vi "SPI Master with debug [Host].vi"() -> ()   [LabVIEW 2019]
uses:
  <vilib>/rvi/interface/RandomDataEmulation/nirviRandomDataOpen.vi
  <vilib>/rvi/interface/common/niFpgaCacheSessionInfoDynamic.vi
  <vilib>/Utility/error.llb/Error Cluster From Error Code.vi
  <vilib>/rvi/errors/niLvFpgaAdjustHostInterfaceError.vi
  <vilib>/Waveform/DWDTOps.llb/DWDT Binary U8 to Digital.vi
  <vilib>/Waveform/DWDTOps.llb/DWDT Binary U32 to Digital.vi
  <vilib>/FPGAPlugInAG/Dynamic/niLvFpga_Close_Dynamic.vi
  <vilib>/rvi/interface/nirviOpenFPGA/nirviOpenFPGA.xnode
  SPI Master with debug [FPGA].vi
  <vilib>/rvi/interface/nirviReadWriteControl/nirviReadWriteControl.xnode
  <vilib>/rvi/interface/nirviMethod/nirviMethod.xnode
  <vilib>/rvi/interface/nirviCloseFPGA/nirviCloseFPGA.xnode
  NiFpgaLv.dll
  <vilib>/rvi/interface/Simulation/niFpgaSimulationCallBeginRW.vi
  <vilib>/FPGAPlugInAG/Dynamic/niLvFpga_ReadFifo_Dynamic.vi
  <vilib>/rvi/errors/niLvFpgaMergeErrorWithErrorCode.vi
panel:
  in  "CPOL":bool
  in  "CPHA":bool
  in  "Data Length":u8=16
  in  "Data In":u32=2779077210 format="%x"
  out "Digital Waveform Graph":digitalwaveform[](graph)=[{"t0"=timestamp(0 s since 1904-01-01), "dt"=1e-08, "Y"={"transitions"=[0, 1, 2, 3, 4, 5, 6, 7, 8, 9, 10, 11, 12, 13, 14, 15, 16, 17, 18, 19, 20, 21, 22, 23, 24, 25, 26, 27, 28, 29, 30, 31, 32, 33, 99], "data"=[[0, 0, 0, 0, 0, 0, 1, 0], [0, 0, 0, 0, 0, 1, 0, 0], [0, 0, 0, 0, 0, 1, 0, 1], [0, 0, 0, 0, 0, 1, 0, 0], [0, 0, 0, 0, 0, 1, 0, 1], [0, 0, 0, 0, 0, 1, 0, 0], [0, 0, 0, 0, 0, 1, 0, 1], [0, 0, 0, 0, 0, 1, 0, 0], [0, 0, 0, 0, 0, 1, 0, 1], [0, 0, 0, 0, 0, 1, 0, 0], [0, 0, 0, 0, 0, 1, 0, 1], [0, 0, 0, 0, 0, 1, 0, 0], [0, 0, 0, 0, 0, 1, 0, 1], [0, 0, 0, 0, 0, 1, 0, 0], [0, 0, 0, 0, 0, 1, 0, 1], [0, 0, 0, 0, 0, 1, 0, 0], [0, 0, 0, 0, 0, 1, 0, 1], [0, 0, 0, 0, 0, 1, 0, 0], [0, 0, 0, 0, 0, 1, 0, 1], [0, 0, 0, 0, 0, 1, 0, 0], [0, 0, 0, 0, 0, 1, 0, 1], [0, 0, 0, 0, 0, 1, 0, 0], [0, 0, 0, 0, 0, 1, 0, 1], [0, 0, 0, 0, 0, 1, 0, 0], [0, 0, 0, 0, 0, 1, 0, 1], [0, 0, 0, 0, 0, 1, 0, 0], [0, 0, 0, 0, 0, 1, 0, 1], [0, 0, 0, 0, 0, 1, 0, 0], [0, 0, 0, 0, 0, 1, 0, 1], [0, 0, 0, 0, 0, 1, 0, 0], [0, 0, 0, 0, 0, 1, 0, 1], [0, 0, 0, 0, 0, 1, 0, 0], [0, 0, 0, 0, 0, 0, 1, 1], [0, 0, 0, 0, 0, 0, 0, 1], [0, 0, 0, 0, 0, 0, 0, 1]]}}, {"t0"=timestamp(0 s since 1904-01-01), "dt"=1e-08, "Y"={"transitions"=[0, 1, 2, 3, 4, 5, 6, 7, 8, 9, 10, 11, 12, 13, 14, 15, 16, 17, 18, 19, 20, 21, 22, 23, 24, 25, 26, 27, 28, 29, 30, 31, 32, 33, 34, 99], "data"=[[0, 0, 0, 0, 1, 0, 0, 0], [0, 0, 1, 0, 0, 0, 0, 0], [0, 0, 1, 1, 0, 0, 0, 0], [0, 0, 0, 0, 0, 0, 0, 0], [0, 0, 0, 1, 0, 0, 0, 0], [0, 0, 1, 0, 0, 0, 0, 0], [0, 0, 1, 1, 0, 0, 0, 0], [0, 0, 0, 0, 0, 0, 0, 0], [0, 0, 0, 1, 0, 0, 0, 0], [0, 0, 0, 0, 0, 0, 0, 0], [0, 0, 0, 1, 0, 0, 0, 0], [0, 0, 1, 0, 0, 0, 0, 0], [0, 0, 1, 1, 0, 0, 0, 0], [0, 0, 0, 0, 0, 0, 0, 0], [0, 0, 0, 1, 0, 0, 0, 0], [0, 0, 1, 0, 0, 0, 0, 0], [0, 0, 1, 1, 0, 0, 0, 0], [0, 0, 1, 0, 0, 0, 0, 0], [0, 0, 1, 1, 0, 0, 0, 0], [0, 0, 0, 0, 0, 0, 0, 0], [0, 0, 0, 1, 0, 0, 0, 0], [0, 0, 1, 0, 0, 0, 0, 0], [0, 0, 1, 1, 0, 0, 0, 0], [0, 0, 0, 0, 0, 0, 0, 0], [0, 0, 0, 1, 0, 0, 0, 0], [0, 0, 0, 0, 0, 0, 0, 0], [0, 0, 0, 1, 0, 0, 0, 0], [0, 0, 1, 0, 0, 0, 0, 0], [0, 0, 1, 1, 0, 0, 0, 0], [0, 0, 0, 0, 0, 0, 0, 0], [0, 0, 0, 1, 0, 0, 0, 0], [0, 0, 1, 0, 0, 0, 0, 0], [0, 0, 1, 1, 0, 0, 0, 0], [0, 0, 1, 0, 0, 0, 0, 0], [0, 0, 1, 0, 1, 0, 0, 0], [0, 0, 1, 0, 1, 0, 0, 0]]}}, {"t0"=timestamp(0 s since 1904-01-01), "dt"=1e-08, "Y"={"transitions"=[0, 1, 3, 5, 7, 9, 11, 13, 15, 17, 19, 21, 23, 25, 27, 29, 31, 99], "data"=[[1, 0, 1, 0, 0, 1, 0, 1, 1, 0, 1, 0, 0, 1, 0, 1, 0, 1, 0, 1, 1, 0, 1, 0, 0, 1, 0, 1, 1, 0, 1, 0], [0, 1, 0, 0, 1, 0, 1, 1, 0, 1, 0, 0, 1, 0, 1, 0, 1, 0, 1, 1, 0, 1, 0, 0, 1, 0, 1, 1, 0, 1, 0, 0], [1, 0, 0, 1, 0, 1, 1, 0, 1, 0, 0, 1, 0, 1, 0, 1, 0, 1, 1, 0, 1, 0, 0, 1, 0, 1, 1, 0, 1, 0, 0, 0], [0, 0, 1, 0, 1, 1, 0, 1, 0, 0, 1, 0, 1, 0, 1, 0, 1, 1, 0, 1, 0, 0, 1, 0, 1, 1, 0, 1, 0, 0, 0, 0], [0, 1, 0, 1, 1, 0, 1, 0, 0, 1, 0, 1, 0, 1, 0, 1, 1, 0, 1, 0, 0, 1, 0, 1, 1, 0, 1, 0, 0, 0, 0, 0], [1, 0, 1, 1, 0, 1, 0, 0, 1, 0, 1, 0, 1, 0, 1, 1, 0, 1, 0, 0, 1, 0, 1, 1, 0, 1, 0, 0, 0, 0, 0, 0], [0, 1, 1, 0, 1, 0, 0, 1, 0, 1, 0, 1, 0, 1, 1, 0, 1, 0, 0, 1, 0, 1, 1, 0, 1, 0, 0, 0, 0, 0, 0, 0], [1, 1, 0, 1, 0, 0, 1, 0, 1, 0, 1, 0, 1, 1, 0, 1, 0, 0, 1, 0, 1, 1, 0, 1, 0, 0, 0, 0, 0, 0, 0, 0], [1, 0, 1, 0, 0, 1, 0, 1, 0, 1, 0, 1, 1, 0, 1, 0, 0, 1, 0, 1, 1, 0, 1, 0, 0, 0, 0, 0, 0, 0, 0, 0], [0, 1, 0, 0, 1, 0, 1, 0, 1, 0, 1, 1, 0, 1, 0, 0, 1, 0, 1, 1, 0, 1, 0, 0, 0, 0, 0, 0, 0, 0, 0, 0], [1, 0, 0, 1, 0, 1, 0, 1, 0, 1, 1, 0, 1, 0, 0, 1, 0, 1, 1, 0, 1, 0, 0, 0, 0, 0, 0, 0, 0, 0, 0, 0], [0, 0, 1, 0, 1, 0, 1, 0, 1, 1, 0, 1, 0, 0, 1, 0, 1, 1, 0, 1, 0, 0, 0, 0, 0, 0, 0, 0, 0, 0, 0, 0], [0, 1, 0, 1, 0, 1, 0, 1, 1, 0, 1, 0, 0, 1, 0, 1, 1, 0, 1, 0, 0, 0, 0, 0, 0, 0, 0, 0, 0, 0, 0, 0], [1, 0, 1, 0, 1, 0, 1, 1, 0, 1, 0, 0, 1, 0, 1, 1, 0, 1, 0, 0, 0, 0, 0, 0, 0, 0, 0, 0, 0, 0, 0, 0], [0, 1, 0, 1, 0, 1, 1, 0, 1, 0, 0, 1, 0, 1, 1, 0, 1, 0, 0, 0, 0, 0, 0, 0, 0, 0, 0, 0, 0, 0, 0, 0], [1, 0, 1, 0, 1, 1, 0, 1, 0, 0, 1, 0, 1, 1, 0, 1, 0, 0, 0, 0, 0, 0, 0, 0, 0, 0, 0, 0, 0, 0, 0, 0], [0, 1, 0, 1, 1, 0, 1, 0, 0, 1, 0, 1, 1, 0, 1, 0, 0, 0, 0, 0, 0, 0, 0, 0, 0, 0, 0, 0, 0, 0, 0, 0], [0, 1, 0, 1, 1, 0, 1, 0, 0, 1, 0, 1, 1, 0, 1, 0, 0, 0, 0, 0, 0, 0, 0, 0, 0, 0, 0, 0, 0, 0, 0, 0]]}}]
  in  "Stop Simulation":bool
  in  "Simulation Steps":u32=100
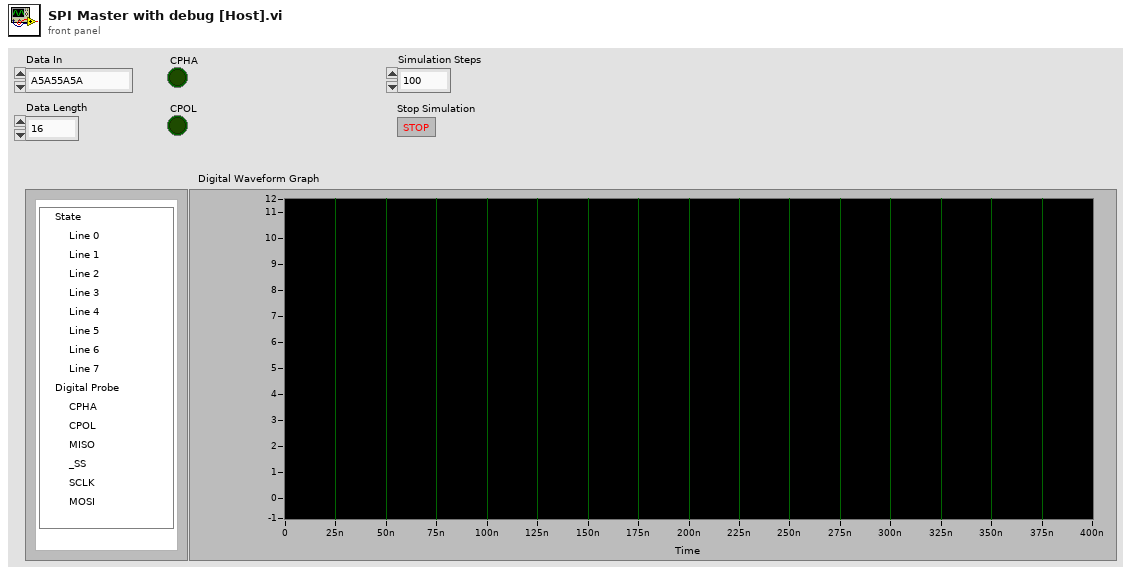
[diagram p1: front panel]
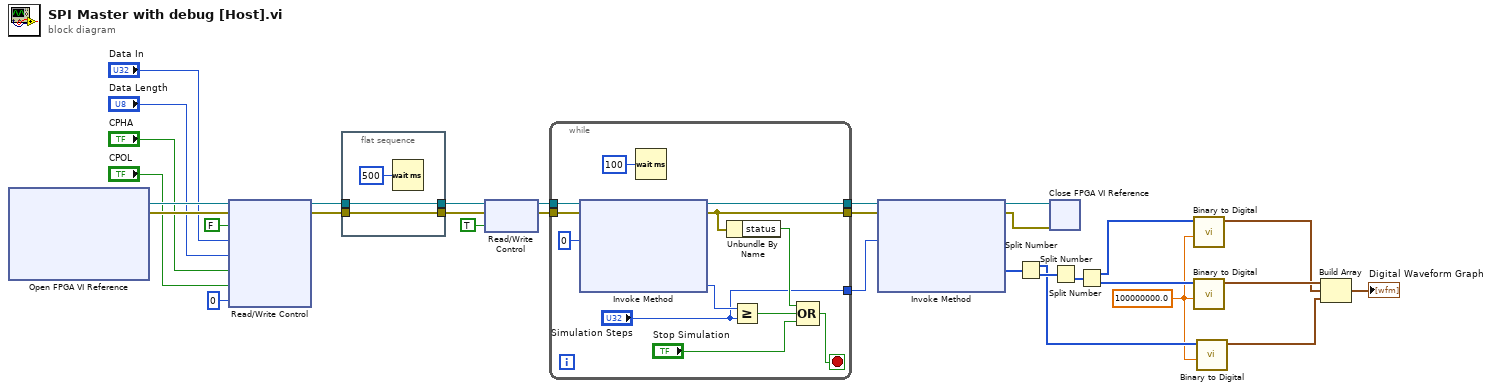
[diagram p0: block diagram]
diagram:
  w5 = 100000000.0 ("sample rate")
  n1 = xnode "Open FPGA VI Reference"() -> ("FPGA VI Reference Out"=w31:refnum<k20>, "error out"=w30:errorcluster)  [unwired: 2 in]
  n2 = xnode "Read/Write Control"("FPGA VI Reference In"=w31, "error in"=w30, "TX"=FALSE, "Data In"="Data In", "Data Length"="Data Length", "CPHA"="CPHA", "CPOL"="CPOL", "HCP-1"=u8 0) -> ("FPGA VI Reference Out"=w3:refnum<k20>, "error out"=w2:errorcluster)
  n3 = flat-sequence {
    tunnel: [w33] -> w29
    tunnel: w3 -> [w33]
    tunnel: w2 -> [w32]
    tunnel: [w32] -> w28
    frame #0 {
      n4 = Wait (ms)(milliseconds to wait=u32 500) -> ()  [unwired: 1 out]
    }
  }
  n5 = xnode "Read/Write Control"("FPGA VI Reference In"=w29, "error in"=w28, "TX"=TRUE) -> ("FPGA VI Reference Out"=w23:refnum<k20>, "error out"=w22:errorcluster)
  n6 = while {
    tunnel: w23 -> [w46]
    tunnel: w22 -> [w45]
    tunnel: [w38] -> w20
    tunnel: [w42] -> w21
    tunnel: ["Simulation Steps"] -> w16
    stop <- w39 stop-if-true
    n7 = xnode "Invoke Method"("FPGA VI Reference In"=w46, "error in"=w45, "Number of Elements"=u32 0) -> ("FPGA VI Reference Out"=w42:refnum<k20>, "error out"=w38:errorcluster, "Elements Remaining"=w36:u32)  [unwired: 1 in, 1 out]
    n8 = Wait (ms)(milliseconds to wait=u32 100) -> ()  [unwired: 1 out]
    n9 = Unbundle By Name(w38) -> ("status"=w37:bool)
    n10 = Greater Or Equal?(x=w36, y="Simulation Steps") -> (x >= y?=w41:bool)
    n11 = Compound Arithmetic op=OR(w37, w41, "Stop Simulation") -> (w39:bool)
  }
  n12 = xnode "Invoke Method"("FPGA VI Reference In"=w21, "error in"=w20, "Number of Elements"=w16) -> ("FPGA VI Reference Out"=w19:refnum<k20>, "error out"=w18:errorcluster, "Data"=w17:u64[])  [unwired: 1 in, 1 out]
  n13 = Split Number(x=w17) -> (hi(x)=w6:u32[], lo(x)=w13:u32[])
  n14 = xnode "Close FPGA VI Reference"("FPGA VI Reference In"=w19, "error in"=w18) -> ()  [unwired: 1 out]
  n15 = Split Number(x=w13) -> (lo(x)=w12:u16[])  [unwired: 1 out]
  n16 = Split Number(x=w12) -> (hi(x)=w14:u8[], lo(x)=w15:u8[])
  n17 = call-poly <vilib>:"Binary to Digital.vi"("sample rate"=w5, "binary array"=w14) -> ("digital waveform"=w10:digitalwaveform)  [unwired: 8 in, 1 out]
  n18 = call-poly <vilib>:"Binary to Digital.vi"("sample rate"=w5, "binary array"=w15) -> ("digital waveform"=w11:digitalwaveform)  [unwired: 8 in, 1 out]
  n19 = call-poly <vilib>:"Binary to Digital.vi"("sample rate"=w5, "binary array"=w6) -> ("digital waveform"=w4:digitalwaveform)  [unwired: 8 in, 1 out]
  n20 = Build Array(w11, w10, w4) -> (→"Digital Waveform Graph":digitalwaveform[])
